vi "slscsl_disconnect.vi"(8 "error in (no error)":errorcluster, 10 "connectionList":string, 11 "slscsl in":refnum<class "slscsl.lvclass">) -> (0 "error out":errorcluster, 2 "SwitchActionsArray":T1 {"RelayAction" items=["CloseRelay"=21, "OpenRelay"=20]}, 3 "slscsl out":refnum<class "slscsl.lvclass">)   [LabVIEW 2015, in "SLSC Switch.lvlib" / "slscsl.lvclass"]
uses:
  slscsl.lvclass
  SwitchActionsArray.ctl
  SwitchAction.ctl
  RelayAction.ctl
  slscsl.lvclass/slscsl.ctl
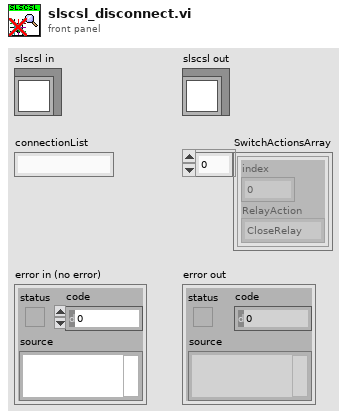
[diagram p1: front panel]
types:
  T1 = typedef "SLSC Switch.lvlib/slscsl.lvclass/SwitchActionsArray.ctl" = T2[]
  T2 = typedef "SLSC Switch.lvlib/slscsl.lvclass/SwitchAction.ctl" = cluster{"index":i32, "RelayAction":T3}
  T3 = typedef "SLSC Switch.lvlib/slscsl.lvclass/RelayAction.ctl" = u32
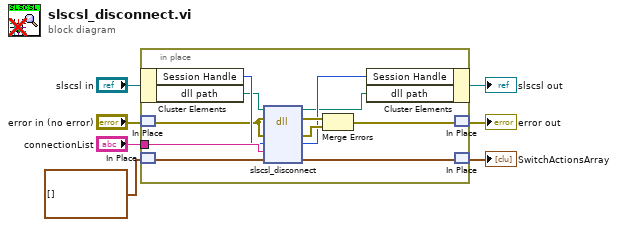
[diagram p0: block diagram]
diagram:
  n1 = in-place {
    in-place-border: "connectionList" -> [w15]
    n2 = in-place-cluster #1("slscsl in") -> ("Session Handle"=w14:u64, "dll path"=w9:path)
    n3 = in-place-match #2("error in (no error)") -> (w13:errorcluster)
    n4 = in-place-match #3(T1 [] ("SwitchActionsArray")) -> (w12:T1)
    n5 = dll-call lib="?" fn="slscsl_disconnect"(path in=w9, error in=w13, "errorCluster"=w13, "sessionHandle"=w14, "dissconnectionList"=w15, "switchActionList"=w12) -> (path out=w8:path, error out=w18:errorcluster, "errorCluster"=w17:errorcluster, "sessionHandle"=w16:u64, "switchActionList"=w11:T1)  [unwired: 3 in]
    n6 = Merge Errors(w18, w17) -> (w10:errorcluster)
    n7 = in-place-cluster #1("Session Handle"=w16, "dll path"=w8) -> (→"slscsl out":refnum<class "slscsl.lvclass">)
    n8 = in-place-match #2(w10) -> (→"error out":errorcluster)
    n9 = in-place-match #3(w11) -> (→"SwitchActionsArray":T1)
  }
